vi "DSF.Engine.Framework.Initialize.Plugins.vi"(8 "error in (no error)":errorcluster, 10 "Plugin Configurations":refnum<class "DSF.Shared.Configuration.Plugin.lvclass">[](array[class]), 11 "Framework in":refnum<class "DSF.Engine.Framework.lvclass">) -> (0 "error out":errorcluster, 2 "Plugins":refnum<class "DSF.Engine.Plugin.lvclass">[](array[class]), 3 "Framework out":refnum<class "DSF.Engine.Framework.lvclass">)   [LabVIEW 2017, in "DSF.Engine.lvlib" / "DSF.Engine.Framework.lvclass"]
uses:
  DSF.Engine.Framework.lvclass
  Plugin/DSF.Engine.Plugin.lvclass
  Shared/Classes/Plugin/DSF.Shared.Configuration.Plugin.lvclass
  Timing/DSF.Engine.Timing.lvclass
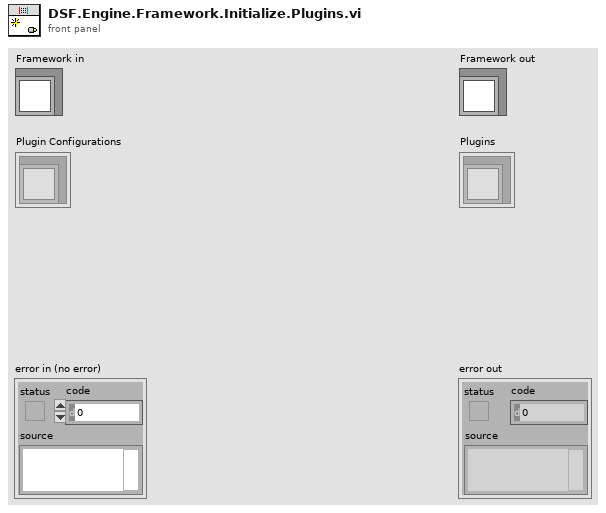
[diagram p1: front panel]
types:
  T1 = typedef "DSF.Shared.lvlib/DSF.Shared.Typedefs.Cycle Timing Factors.ctl" = cluster{"Priority":u64, "Decimation":u64, "Offset":u64}
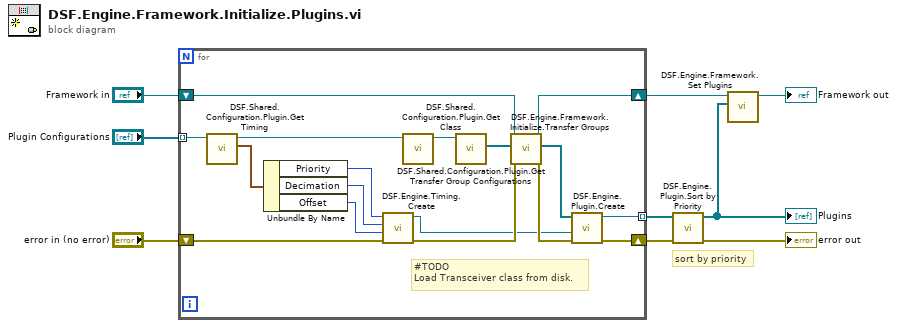
[diagram p0: block diagram]
diagram:
  # "sort by priority"
  n1 = for {
    shift-right: [w20] -> w7
    shift-left: "error in (no error)" -> [w21]
    shift-right: [w15] -> w3
    shift-left: "Framework in" -> [w16]
    tunnel: "Plugin Configurations" -> [w26] mode=indexing
    tunnel: [w11] -> w2 mode=indexing
    # "#TODO\nLoad Transceiver class from disk."
    n2 = call "DSF.Shared.Configuration.Plugin.Get Timing.vi"("Plugin Configuration in"=w26) -> ("cycle timing"=w25:T1, "Plugin Configuration out"=w19:refnum<class "DSF.Shared.Configuration.Plugin.lvclass">)  [unwired: 9 in]
    n3 = Unbundle By Name(w25) -> ("Priority"=w22:u64, "Decimation"=w23:u64, "Offset"=w24:u64)
    n4 = call "DSF.Engine.Timing.Create.vi"("error in (no error)"=w21, "Offset"=w24, "Decimation"=w23, "Priority"=w22) -> ("error out"=w13:errorcluster, "Timing"=w10:refnum<class "DSF.Engine.Timing.lvclass">)  [unwired: 6 in]
    n5 = call "DSF.Shared.Configuration.Plugin.Get Class.vi"("Plugin Configuration in"=w19) -> ("Plugin Configuration out"=w18:refnum<class "DSF.Shared.Configuration.Plugin.lvclass">)  [unwired: 9 in, 1 out]
    n6 = call "DSF.Shared.Configuration.Plugin.Get Transfer Group Configurations.vi"("Plugin Configuration in"=w18) -> ("Transfer Group Configurations"=w17:refnum<class "DSF.Shared.Configuration.Transfer Group.lvclass">[])  [unwired: 9 in, 1 out]
    n7 = call "DSF.Engine.Framework.Initialize.Transfer Groups.vi"("error in (no error)"=w13, "Transfer Group Configurations"=w17, "Framework in"=w16) -> ("error out"=w12:errorcluster, "Transfer Groups"=w14:refnum<class "DSF.Engine.Transfer Group.lvclass">[], "Framework out"=w15:refnum<class "DSF.Engine.Framework.lvclass">)  [unwired: 6 in]
    n8 = call "DSF.Engine.Plugin.Create.vi"("error in (no error)"=w12, "Timing"=w10, "Transfer Groups"=w14) -> ("error out"=w20:errorcluster, "Plugin out"=w11:refnum<class "DSF.Engine.Plugin.lvclass">)  [unwired: 7 in]
  }
  n9 = call "DSF.Engine.Plugin.Sort by Priority.vi"("error in (no error)"=w7, "Plugins in"=w2) -> ("error out"=→"error out":errorcluster, "Plugins out"=w1:refnum<class "DSF.Engine.Plugin.lvclass">[])  [unwired: 8 in]
  "Plugins" <- w1
  n10 = call "DSF.Engine.Framework.Set Plugins.vi"("Plugins"=w1, "Framework in"=w3) -> ("Framework out"=→"Framework out":refnum<class "DSF.Engine.Framework.lvclass">)  [unwired: 9 in]
